vi "Read from Port.vi"(8 "error in":errorcluster, 10 "TEC Cmd":T1, 11 "TE Cooler in":refnum<class "TE Cooler.lvclass">=refnum) -> (0 "error out":errorcluster, 1 "outputStr":string, 2 "scaledOut":sgl, 3 "TE Cooler out":refnum<class "TE Cooler.lvclass">)   [LabVIEW 2014, in "TE Cooler.lvlib" / "TE Cooler.lvclass"]
doc: "Send a command and read the resulting data out. From the manual:\n\nTo write a command to the controller, the controlling computer must send the following ASCII characters:\n(stx)00CCDDDDDDDDSS(etx)\n\nHere, 00 is the only acceptable address for the TC-36-25; CC are the command characters; DDDDDDDD is the ASCII representation of the hexadecimal return or send value. Negative numbers are represented by the hex 2fs complement of the number (32-bit word size):\n 1base10 = 0000000116\n-1base10=ffffffff16"
uses:
  TE Cooler.lvclass
  Controls/Command.ctl
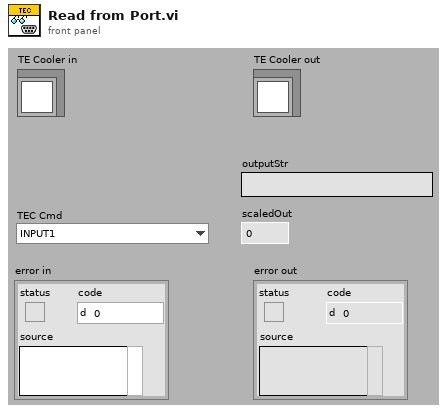
[diagram p1: front panel]
types:
  T1 = typedef "TE Cooler.lvlib/TE Cooler.lvclass/Command.ctl" = enum16{"INPUT1", "DESIRED CONTROL VALUE", "POWER OUTPUT", "ALARM STATUS", "INPUT 2", "OUTPUT CURRENT COUNTS", "ALARM TYPE", "SET TYPE DEFINE", "SENSOR TYPE", "CONTROL TYPE", "CONTROL OUTPUT POLARITY", "POWER ON/OFF", "OUTPUT SHUTDOWN IF ALARM", "FIXED DESIRED CONTROL SETTING", "PROPORTIONAL BANDWIDTH", "INTEGRAL GAIN", "DERIVATIVE GAIN", "LOW EXTERNAL SET RANGE", "HIGH EXTERNAL SET RANGE", "ALARM DEADBAND", "HIGH ALARM SETTING", "LOW ALARM SETTING", "CONTROL DEADBAND SETTING", "INPUT1 OFFSET", "INPUT2 OFFSET", "HEAT MULTIPLIER", "COOL MULTIPLIER", "OVER CURRENT COUNT COMPARE VALUE", "ALARM LATCH ENABLE", "NOT USED", "ALARM LATCH RESET", "CHOOSE SENSOR FOR ALARM FUNCTION", "CHOOSE TEMPERATURE WORKING UNITS", "EEPROM WRITE ENABLE", "OVER CURRENT CONTINUOUS", "OVER CURRENT RESTART ATTEMPTS", "JP3 DISPLAY ENABLE"}
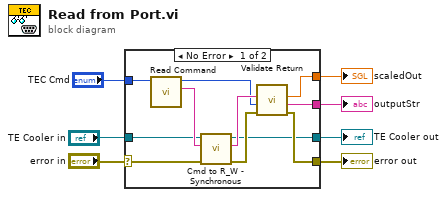
[diagram p0: block diagram]
diagram:
  n1 = case shown="No Error" "error in" {
    selector: "error in" -> [w12 w20]
    tunnel: [w14 w20] -> w6
    tunnel: [w11 w19] -> w4
    tunnel: "TE Cooler in" -> [w13 w19]
    tunnel: [w10 _] -> w3
    tunnel: [w9 _] -> w2
    tunnel: "TEC Cmd" -> [w8 _]
    frame No Error {
      n2 = call "Read Command.vi"("TEC Cmd"=w8) -> ("String"=w18:string, "Numeric"=w15:i32)  [unwired: 9 in]
      n3 = call-dynamic "Cmd to R_W - Synchronous.vi"("error in"=w12, "write buffer"=w18, "Serial IO in"=w13) -> ("error out"=w16:errorcluster, "read buffer"=w17:string, "Serial IO out"=w11:refnum<class "TE Cooler.lvclass">)  [unwired: 6 in]
      n4 = call "Validate Return.vi"("error in"=w16, "Divisor"=w15, "Rtn Str"=w17) -> ("error out"=w14:errorcluster, "outputStr"=w9:string, "Output Value"=w10:sgl)  [unwired: 6 in]
    }
    frame Error {
    }
  }
  "error out" <- w6
  "TE Cooler out" <- w4
  "scaledOut" <- w3
  "outputStr" <- w2
